vi "Init Inline State Variables.vi"(8 "error in":errorcluster, 11 "Device Reference in":T7 format="%.0x") -> (0 "error out":errorcluster, 3 "State Vars":T1 {"CompiledSettings"."Result Ch Data Refs" format="%.0x"; "CompiledSettings"."Parameter Block Data Refs"."Data Reference" format="%.0x"})   [LabVIEW 2014, in "Waveform-Processing-Custom-Device Engine.lvlib"]
uses:
  Waveform-Processing-Custom-Device Engine.lvlib
  <vilib>/NI Veristand/Custom Device API/Custom Device Item Ref.ctl
  Types/Inline State Vars.ctl
  Types/Async FIFOs.ctl
  Shared/CompiledSettings.ctl
  <vilib>/NI Veristand/Custom Device API/Block Data Reference.ctl
  <vilib>/NI Veristand/Custom Device API/Data Reference.ctl
  <vilib>/NI Veristand/Custom Device API/Waveform Data Reference.ctl
  Shared/Constants.vi
  <vilib>/NI Veristand/Custom Device API/Get Item Property (Variant).vi
  Shared/Waveform-Processing-Custom-Device Shared.lvlib
  <vilib>/NI Veristand/Custom Device API/Custom Device API.lvlib
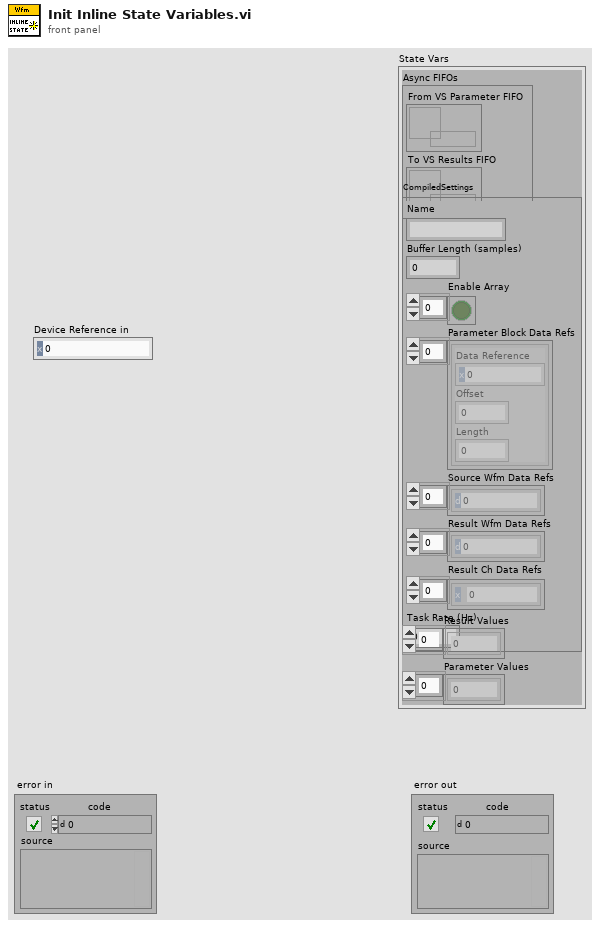
[diagram p1: front panel]
types:
  T1 = typedef "Waveform-Processing-Custom-Device Engine.lvlib/Inline State Vars.ctl" = cluster{"Async FIFOs":T2, "CompiledSettings":T3, "Result Values":dbl[], "Parameter Values":dbl[]}
  T2 = typedef "Waveform-Processing-Custom-Device Engine.lvlib/Async FIFOs.ctl" = cluster{"From VS Parameter FIFO":refnum<k33>, "To VS Results FIFO":refnum<k33>}
  T3 = typedef "Waveform-Processing-Custom-Device Shared.lvlib/CompiledSettings.ctl" = cluster{"Name":string, "Buffer Length (samples)":u32, "Enable Array":bool[], "Parameter Block Data Refs":T4[], "Source Wfm Data Refs":T6[], "Result Wfm Data Refs":T6[], "Result Ch Data Refs":T5[], "Task Rate (Hz)":dbl}
  T4 = typedef "Custom Device API.lvlib/Block Data Reference.ctl" = cluster{"Data Reference":T5, "Offset":i32, "Length":i32}
  T5 = typedef "Custom Device API.lvlib/Data Reference.ctl" = i32
  T6 = typedef "Custom Device API.lvlib/Waveform Data Reference.ctl" = i32
  T7 = typedef "Custom Device API.lvlib/Custom Device Item Ref.ctl" = u64
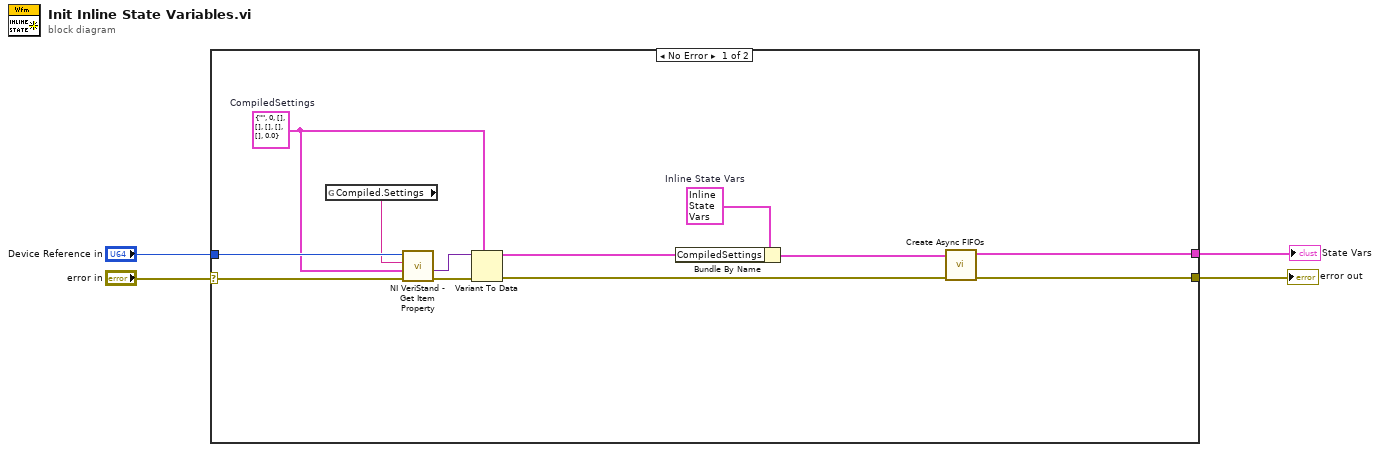
[diagram p0: block diagram]
diagram:
  n1 = case shown="No Error" "error in" {
    selector: "error in" -> [w15 w17]
    tunnel: [w14 w17] -> w3
    tunnel: "Device Reference in" -> [w16 _]
    tunnel: [w12 _] -> w1
    frame No Error {
      w5 = T3 {"Name"="", "Buffer Length (samples)"=0, "Enable Array"=[], "Parameter Block Data Refs"=[], "Source Wfm Data Refs"=[], "Result Wfm Data Refs"=[], "Result Ch Data Refs"=[], "Task Rate (Hz)"=0.0}  # CompiledSettings
      w13 = T1 {"Async FIFOs"={"From VS Parameter FIFO"=refnum, "To VS Results FIFO"=refnum}, "CompiledSettings"={"Name"="", "Buffer Length (samples)"=0, "Enable Array"=[], "Parameter Block Data Refs"=[], "Source Wfm Data Refs"=[], "Result Wfm Data Refs"=[], "Result Ch Data Refs"=[], "Task Rate (Hz)"=0.0}, "Result Values"=[], "Parameter Values"=[]}  # Inline State Vars
      n2 = global read "Constants.vi" "Compiled.Settings"() -> (w10:string)
      n3 = call-poly <vilib>:"NI VeriStand - Get Item Property.vi"("error in (no error)"=w15, "Default Value"=w5, "Property Name"=w10, "Item Ref in"=w16) -> ("error out"=w9:errorcluster, "Value"=w8:variant)  [unwired: 4 in, 2 out]
      n4 = Variant To Data(error in=w9, type=w5, Variant=w8) -> (data=w11:T3, error out=w7:errorcluster)
      n5 = Bundle By Name(cluster=w13, "CompiledSettings"=w11) -> (w6:T1)
      n6 = call "Create Async FIFOs.vi"("error in (no error)"=w7, "State Vars"=w6) -> ("error out"=w14:errorcluster, "State Vars out"=w12:T1)  [unwired: 8 in]
    }
    frame Error {
    }
  }
  "error out" <- w3
  "State Vars" <- w1
